vi "Tree to String Array.vi"(7 "Level":i32, 9 "Delimiter (Tab)":string="\t", 11 "Tree in":variant) -> (3 "String Array":string[](array[string]))   [LabVIEW 2023, in "VIDoc Printer.lvlib" / "VIDoc Printer.lvclass"]
uses:
  VIDoc Printer.lvclass
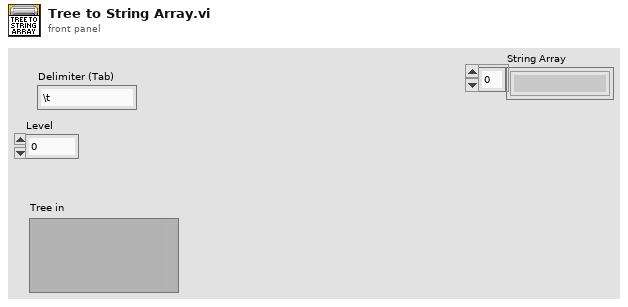
[diagram p1: front panel]
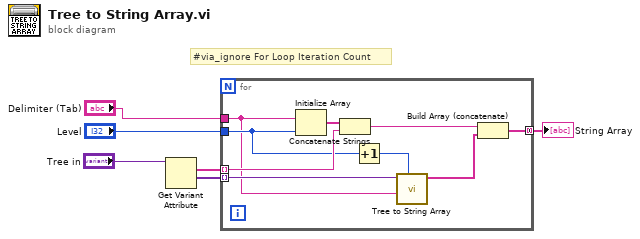
[diagram p0: block diagram]
diagram:
  # "#via_ignore For Loop Iteration Count"
  n1 = Get Variant Attribute(Variant="Tree in") -> (names=w5:string[], values=w4:variant[])  [unwired: 3 in, 2 out]
  n2 = for {
    tunnel: w5 -> [w13] mode=indexing
    tunnel: w4 -> [w15] mode=indexing
    tunnel: "Level" -> [w9]
    tunnel: [w11] -> w2 mode=concatenating
    tunnel: "Delimiter (Tab)" -> [w7]
    n3 = Initialize Array(w7, w9) -> (w14:string[])
    n4 = Concatenate Strings(w14, w13) -> (w12:string)
    n5 = Increment(x=w9) -> (x+1=w8:i32)
    n6 = call "Tree to String Array.vi"("Level"=w8, "Delimiter (Tab)"=w7, "Tree in"=w15) -> ("String Array"=w10:string[])  [unwired: 8 in]
    n7 = Build Array (concatenate)(w12, w10) -> (w11:string[])
  }
  "String Array" <- w2
